vi "XY Graph Get Plot Data Point at Mouse.vi"(8 "Error In":errorcluster, 9 "Excluded Plots":i32[](array[numeric]), 10 "Coords":T1, 11 "XYGraph in":refnum<vi>) -> (0 "Error Out":errorcluster, 1 "Point  Index":i32, 2 "Plot Number":i32, 3 "Plot Data Point":cluster{"X":dbl, "Y":dbl}, 4 "Distance to Plot":dbl)   [LabVIEW 2021, in "XY Graph Add-Ons.lvlib"]
uses:
  XY Graph Add-Ons.lvlib
  <vilib>/Utility/miscctls.llb/LVPoint32TypeDef.ctl
  Get Plot at Mouse Click (XY Graph)/Get Plot at Mouse Click [AAC].vi
  Graphs.lvlib
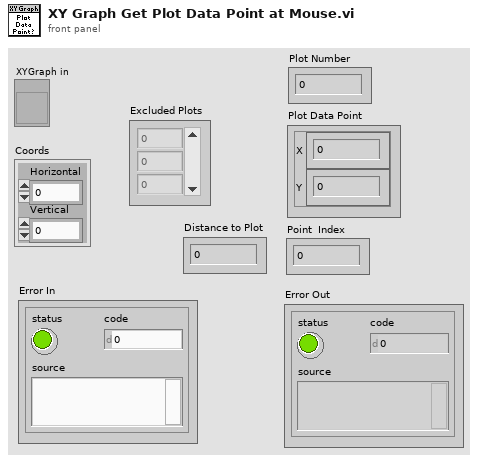
[diagram p1: front panel]
types:
  T1 = typedef "LVPoint32TypeDef.ctl" = cluster{"Horizontal":i32, "Vertical":i32}
  T2 = typedef "XY Graph Add-Ons.lvlib/XY Graph Refnum.ctl" = refnum<vi>
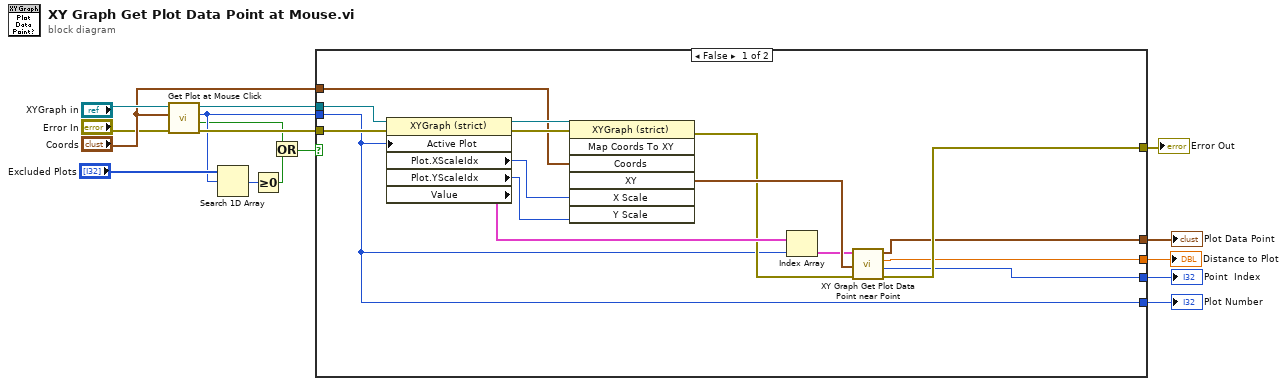
[diagram p0: block diagram]
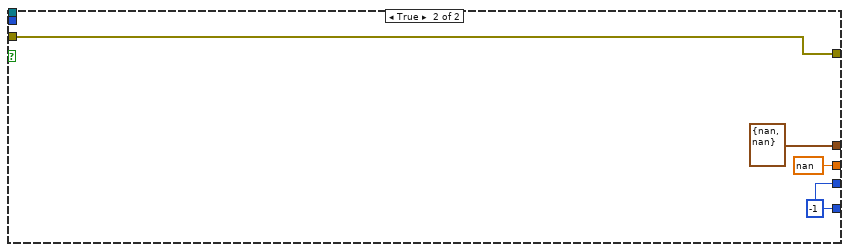
[diagram p2: hidden frame]
diagram:
  n1 = call-poly "Get Plot at Mouse Click.vi"("error in (no error)"="Error In", "Mouse Click Coordinates"="Coords", "XYGraph Ref"="XYGraph in") -> ("error out"=w11:errorcluster, "Click is in Legend?"=w2:bool, "Plot at Coordinates"=w5:i32, "XYGraph Ref"=w12:T2)  [unwired: 2 in, 3 out]
  n2 = Search 1D Array(1D array="Excluded Plots", element=w5) -> (index of element=w4:i32)  [unwired: 1 in]
  n3 = Greater Or Equal To 0?(x=w4) -> (x >= 0?=w1:bool)
  n4 = Or(x=w2, y=w1) -> (x .or. y?=w3:bool)
  n5 = case shown="False" w3 {
    tunnel: [w25 w36] -> w16
    tunnel: "Coords" -> [w23 _]
    tunnel: w12 -> [w22 _]
    tunnel: w11 -> [w21 w36]
    tunnel: w5 -> [w17 _]
    tunnel: [w20 cluster{"X":dbl, "Y":dbl} {"X"=nan, "Y"=nan} ("Plot Data Point")] -> w10
    tunnel: [w19 w35] -> w9
    tunnel: [w18 nan ("Distance to Plot")] -> w8
    tunnel: [w17 w35] -> w7
    frame False {
      n6 = property class="XYGraph (strict)"(reference=w22, error in=w21, "Active Plot"=w17) -> (reference out=w32:T2, error out=w31:errorcluster, "Plot.XScaleIdx"=w30:u32, "Plot.YScaleIdx"=w29:u32, "Value"=w28:cluster{"X Array":dbl[], "Y Array":dbl[]}[])
      n7 = invoke class="XYGraph (strict)" method="Map Coords To XY"(reference=w32, error in=w31, "Coords"=w23, "X Scale"=w30, "Y Scale"=w29) -> (error out=w26:errorcluster, "XY"=w27:cluster{"X":dbl, "Y":dbl})  [unwired: 2 in, 5 out]
      n8 = Index Array(array=w28, index=w17) -> (element=w24:cluster{"X Array":dbl[], "Y Array":dbl[]})
      n9 = call "XY Graph Get Plot Data Point near Point.vi"("Error In"=w26, "Point"=w27, "Plot in"=w24) -> ("Error Out"=w25:errorcluster, "Point  Index"=w19:i32, "Distance to Plot"=w18:dbl, "Plot Data Point"=w20:cluster{"X":dbl, "Y":dbl})  [unwired: 5 in]
    }
    frame True {
      w35 = -1 ("Plot at Coordinates")
    }
  }
  "Error Out" <- w16
  "Distance to Plot" <- w8
  "Point  Index" <- w9
  "Plot Number" <- w7
  "Plot Data Point" <- w10
